vi "求水仙花数.vi"() -> (3 "水仙花数":i32[](array[numeric]))   [LabVIEW 2011]
doc: "功能：\n\n求三位数中的水仙花数\n\n水仙花数的定义：\n\n所谓水仙花数，是指一个三位数，其各个位数的立方和等于该数本身，比如：\n\n153=1^3+5^+3^\n\ncsxcs_366创建"
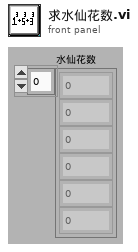
[diagram p1: front panel]
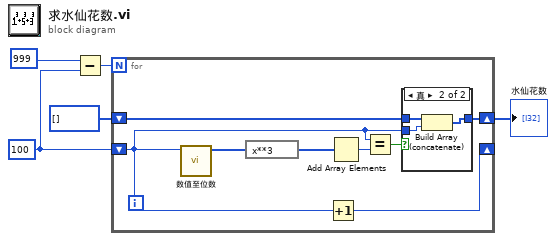
[diagram p0: block diagram]
diagram:
  w3 = 100
  n1 = Subtract(x=999, y=w3) -> (x-y=w4:i32)
  n2 = for {
    N: w4 -> [_]
    shift-right: [w8] -> _
    shift-left: w3 -> [w9]
    shift-right: [w6] -> w1
    shift-left: i32[] [] -> [w7]
    n3 = call-poly "数值至位数.vi"("输入数值"=w9) -> ("位数数组"=w13:i32[])  [unwired: 9 in, 1 out]
    n4 = expression code="x**3"(w13) -> (w12:i32[])
    n5 = Increment(x=w9) -> (x+1=w8:i32)
    n6 = Add Array Elements(numeric array=w12) -> (sum=w11:i32)
    n7 = Equal?(x=w9, y=w11) -> (x = y?=w10:bool)
    n8 = case shown="真" w10 {
      tunnel: w7 -> [w14 w15]
      tunnel: [w14 w16] -> w6
      tunnel: w9 -> [_ w17]
      frame False {
      }
      frame True {
        n9 = Build Array (concatenate)(w15, w17) -> (w16:i32[])
      }
    }
  }
  "水仙花数" <- w1
